vi "FGV_Macro Settings to GFG.vi"(7 "FGV_Macro Settings to GFG_Command":T3, 8 "error in (no error)":errorcluster, 9 "Source VI":string, 10 "New Settings IN":T2[](array[typedef]), 11 "Settings type string IN":string) -> (0 "error out":errorcluster, 2 "Backed up variable name":string, 3 "Current Settings OUT":T2[](array[typedef]))   [LabVIEW 2012]
doc: "SciScan 1.2 160622\nThis VI controls the bidirectional communication between macro scan settings and the GFG .\n\nThe implemented functioinalities include backing up current settings, over-writing the GFG values with new values and restoring backed up settings to the GFG"
uses:
  Custom Controls and Typedefs/GFG Variable for IO.ctl
  FGV_Macro Settings to GFG_Command.ctl
  Custom Controls/Setting File Types.ctl
panel:
  in  "Setting File Type IN":T1=enum."Configuration Settings"
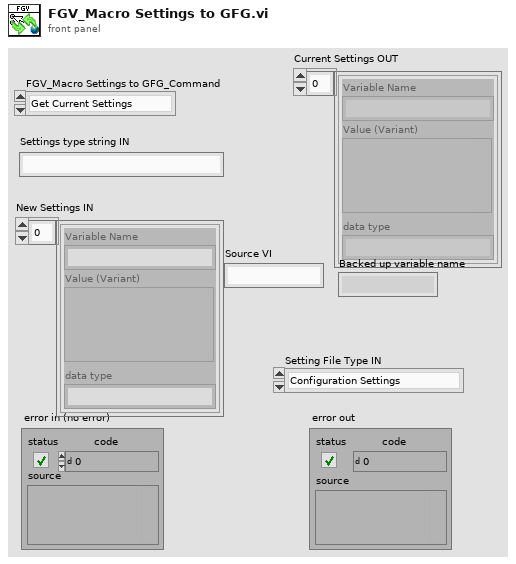
[diagram p1: front panel]
types:
  T1 = typedef "Setting File Types.ctl" = enum16{"2D.Frame.Scan.Settings", "2D.Line.Scan.Settings", "Z.Stack.Settings", "HW Settings", "Configuration Settings", "Unknown Settings", "Fast.Z.Settings"}
  T2 = typedef "GFG Variable for IO.ctl" = cluster{"Variable Name":string, "Value (Variant)":variant, "data type":string}
  T3 = typedef "FGV_Macro Settings to GFG_Command.ctl" = enum16{"Get Current Settings", "Backup Curent Settings", "Recover Backed up settings", "Overwrite Current Settings"}
  T4 = enum16{"Get Settings Table ", "Read Settings File", "Get Specified Settings"}
  T5 = typedef "VariantType.lvlib/Type.ctl" = enum8{"Invalid Type", "Void", "I8", "I16", "I32", "I64", "U8", "U16", "U32", "U64", "Single Float", "Double Float", "Extended Float", "Single Complex", "Double Complex", "Extended Complex", "Enum U8", "Enum U16", "Enum U32", "Enum U64", "Single Float With Unit", "Double Float With Unit", "Extended Float With Unit", "Single Complex with Unit", "Double Complex with Unit", "Extended Complex with Unit", "Boolean", "String", "Path", "Picture", "Tag", "Array", "Cluster", "Variant", "LV Variant", "Waveform", "Timestamp", "Digital Waveform", "Digital Data", "ExpressData", "Refnum", "External Data", "VI", "Poly VI", "LabVIEW Class Instance", "Fixed Point"}
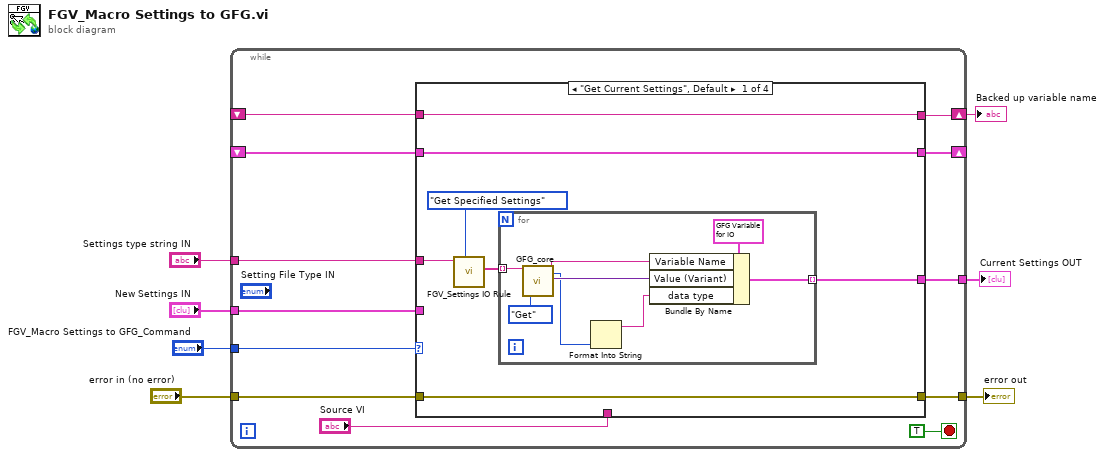
[diagram p0: block diagram]
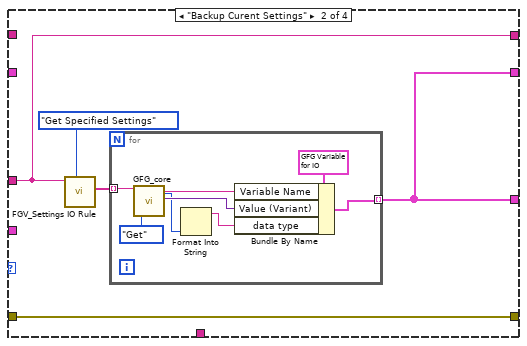
[diagram p2: hidden frame]
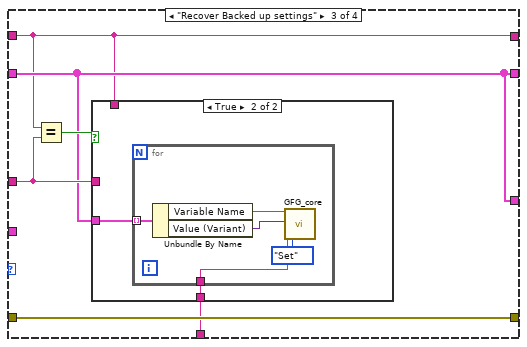
[diagram p3: hidden frame]
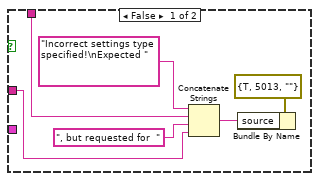
[diagram p4: hidden frame]
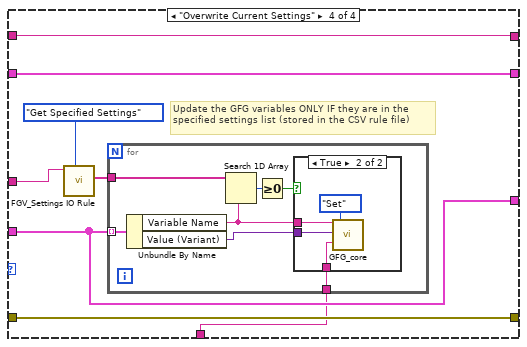
[diagram p5: hidden frame]
diagram:
  n1 = while {
    tunnel: "FGV_Macro Settings to GFG_Command" -> [w19]
    tunnel: "Settings type string IN" -> [w17]
    shift-right: [w16] -> _
    shift-left: _ -> [w15]
    shift-right: [w14] -> w5
    shift-left: _ -> [w13]
    tunnel: [w12] -> w4
    tunnel: [w11] -> w3
    tunnel: "error in (no error)" -> [w10]
    tunnel: "New Settings IN" -> [w9]
    stop <- TRUE stop-if-true
    n2 = case shown="\"Get Current Settings\", Default" w19 {
      tunnel: w17 -> [w22 w37 w52 w72]
      tunnel: [w25 w35 w51 w70] -> w16
      tunnel: w15 -> [w25 _ w51 w70]
      tunnel: [w26 w37 w50 w69] -> w14
      tunnel: w13 -> [w26 _ w50 w69]
      tunnel: [w21 w35 w51 w68] -> w12
      tunnel: [w20 w36 w49 w74] -> w11
      tunnel: w10 -> [w20 w36 w49 w74]
      tunnel: w9 -> [_ _ _ w68]
      tunnel: "Source VI" -> [_ _ w48 w67]
      frame "Get Current Settings", Default {
        n3 = call "FGV_Settings IO Rule.vi"("Command_Settings IO Rule"=T4."Get Specified Settings", "Settings Type IN"=w22) -> ("Specified Settings (OUT)"=w23:string[])  [unwired: 7 in, 2 out]
        n4 = for {
          tunnel: w23 -> [w34] mode=indexing
          tunnel: [w29] -> w21 mode=indexing
          n5 = call "GFG_core.vi"("Variable Name in"=w34, "Action"=enum16{"Init", "Set", "Get", "Clear"}."Get") -> ("Variable Name Out"=w31:string, "Data Type Out"=w28:T5, "Variant Out"=w30:variant)  [unwired: 11 in, 4 out]
          n6 = Format Into String(w28) -> (resulting string=w27:string)  [unwired: 3 in, 1 out]
          n7 = Bundle By Name(cluster=T2 {"Variable Name"="", "Value (Variant)"=variant, "data type"=""} ("GFG Vairable for IO"), "Variable Name"=w31, "Value (Variant)"=w30, "data type"=w27) -> (w29:T2)
        }
      }
      frame "Backup Curent Settings" {
        n8 = call "FGV_Settings IO Rule.vi"("Command_Settings IO Rule"=T4."Get Specified Settings", "Settings Type IN"=w37) -> ("Specified Settings (OUT)"=w38:string[])  [unwired: 7 in, 2 out]
        n9 = for {
          tunnel: w38 -> [w47] mode=indexing
          tunnel: [w42] -> w35 mode=indexing
          n10 = call "GFG_core.vi"("Variable Name in"=w47, "Action"=enum16{"Init", "Set", "Get", "Clear"}."Get") -> ("Variable Name Out"=w44:string, "Data Type Out"=w41:T5, "Variant Out"=w43:variant)  [unwired: 11 in, 4 out]
          n11 = Format Into String(w41) -> (resulting string=w40:string)  [unwired: 3 in, 1 out]
          n12 = Bundle By Name(cluster=T2 {"Variable Name"="", "Value (Variant)"=variant, "data type"=""} ("GFG Vairable for IO"), "Variable Name"=w44, "Value (Variant)"=w43, "data type"=w40) -> (w42:T2)
        }
      }
      frame "Recover Backed up settings" {
        n13 = Equal?(x=w50, y=w52) -> (x = y?=w53:bool)
        n14 = case shown="True" w53 {
          tunnel: w52 -> [w54 _]
          tunnel: w51 -> [_ w61]
          tunnel: w50 -> [w56 _]
          tunnel: w48 -> [_ w60]
          frame False {
            n15 = Concatenate Strings("Incorrect settings type specified!\nExpected " ("source"), w56, ", but requested for  " ("source"), w54) -> (w58:string)
            n16 = Bundle By Name(cluster=errorcluster {"status"=TRUE, "code"=5013, "source"=""} ("error constant"), "source"=w58) -> ()  [unwired: 1 out]
          }
          frame True {
            n17 = for {
              tunnel: w61 -> [w65] mode=indexing
              tunnel: w60 -> [w62]
              n18 = Unbundle By Name(w65) -> ("Variable Name"=w64:string, "Value (Variant)"=w63:variant)
              n19 = call "GFG_core.vi"("Variable Name in"=w64, "Variant in"=w63, "Source VI"=w62, "Action"=enum16{"Init", "Set", "Get", "Clear"}."Set") -> ()  [unwired: 9 in, 7 out]
            }
          }
        }
      }
      frame "Overwrite Current Settings" {
        # "Update the GFG variables ONLY IF they are in the specified settings list (stored in the CSV rule file)"
        n20 = call "FGV_Settings IO Rule.vi"("Command_Settings IO Rule"=T4."Get Specified Settings", "Settings Type IN"=w72) -> ("Specified Settings (OUT)"=w71:string[])  [unwired: 7 in, 2 out]
        n21 = for {
          tunnel: w71 -> [w81]
          tunnel: w68 -> [w80] mode=indexing
          tunnel: w67 -> [w75]
          n22 = Unbundle By Name(w80) -> ("Variable Name"=w77:string, "Value (Variant)"=w76:variant)
          n23 = Search 1D Array(1D array=w81, element=w77) -> (index of element=w79:i32)  [unwired: 1 in]
          n24 = Greater Or Equal To 0?(x=w79) -> (x >= 0?=w78:bool)
          n25 = case shown="True" w78 {
            tunnel: w77 -> [_ w84]
            tunnel: w76 -> [_ w83]
            tunnel: w75 -> [_ w82]
            frame False {
            }
            frame True {
              n26 = call "GFG_core.vi"("Variable Name in"=w84, "Variant in"=w83, "Source VI"=w82, "Action"=enum16{"Init", "Set", "Get", "Clear"}."Set") -> ()  [unwired: 9 in, 7 out]
            }
          }
        }
      }
    }
  }
  "error out" <- w3
  "Current Settings OUT" <- w4
  "Backed up variable name" <- w5
